vi "RSZVB Get Logical Port Common Ref Impedance.vi"(8 "error in (no error)":errorcluster {"code" format="%.0x"}, 9 "Port (1)":i32=1, 10 "Channel (1)":i32=1, 11 "VISA session":refnum<visa-resource-name>) -> (0 "error out":errorcluster {"code" format="%.0x"}, 1 "Imaginary":dbl format="%^.3e", 2 "Real":dbl format="%^.3e", 3 "dup VISA session":refnum<visa-resource-name>)   [LabVIEW 2011]
doc: "This VI returns the complex common mode reference impedance for the balanced (logical) port numbered <log_port>. \n\nRemote-control command(s):\n[SENSe<Ch>:]LPORt<log_port>:ZCOMmon?"
uses:
  _utility/RSZVB Global Data.vi
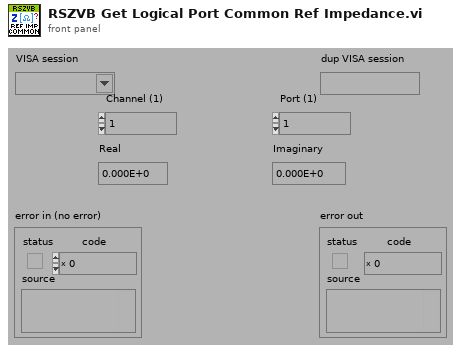
[diagram p1: front panel]
types:
  T1 = cluster{"Error Checking (T: On)":bool, "Installed Options":string[], "Data Valid?":bool, "Ports":i32, "Model":string[], "Option Checking (T: On)":bool}[]
  T2 = cluster{"Error Checking (T: On)":bool, "Installed Options":string[], "Data Valid?":bool, "Ports":i32, "Model":string[], "Option Checking (T: On)":bool}
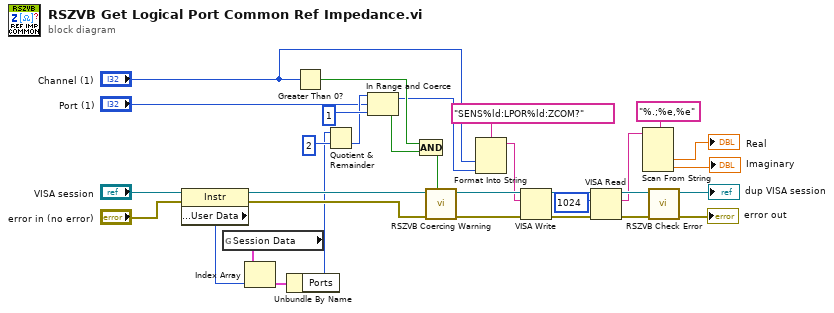
[diagram p0: block diagram]
diagram:
  n1 = property class="Instr"(reference="VISA session", error in="error in (no error)") -> (reference out=w31:refnum<visa-resource-name>, error out=w30:errorcluster, "General Settings:User Data"=w29:u32)
  n2 = global read "RSZVB Global Data.vi" "Session Data"() -> (w28:T1)
  n3 = Index Array(array=w28, index=w29) -> (element=w27:T2)
  n4 = Unbundle By Name(w27) -> ("Ports"=w23:i32)
  n5 = Greater Than 0?(x="Channel (1)") -> (x > 0?=w26:bool)
  n6 = Quotient & Remainder(x=w23, y=2) -> (floor(x/y)=w22:i32)  [unwired: 1 out]
  n7 = In Range and Coerce(upper limit=w22, x="Port (1)", lower limit=1) -> (coerced(x)=w16:i32, In Range?=w21:bool)
  n8 = Compound Arithmetic op=AND(w26, w21) -> (w25:bool)
  n9 = call "RSZVB Coercing Warning.vi"("In Range?"=w25, "error in (no error)"=w30, "VISA session"=w31) -> ("error out"=w20:errorcluster, "dup VISA session"=w19:refnum<visa-resource-name>)  [unwired: 7 in]
  n10 = Format Into String(format string="SENS%ld:LPOR%ld:ZCOM?", "Channel (1)", w16) -> (resulting string=w18:string)  [unwired: 2 in, 1 out]
  n11 = VISA Write(VISA resource name=w19, write buffer=w18, error in (no error)=w20) -> (VISA resource name out=w5:refnum<visa-resource-name>, error out=w6:errorcluster)  [unwired: 1 out]
  n12 = VISA Read(VISA resource name=w5, byte count=u32 1024 ("byte count (0)"), error in (no error)=w6) -> (VISA resource name out=w10:refnum<visa-resource-name>, read buffer=w7:string, error out=w9:errorcluster)  [unwired: 1 out]
  n13 = Scan From String(format string="%.;%e,%e", input string=w7) -> (output 1=→"Real":dbl, output 2=→"Imaginary":dbl)  [unwired: 4 in, 3 out]
  n14 = call "RSZVB Check Error.vi"("error in (no error)"=w9, "VISA session"=w10) -> ("error out"=→"error out":errorcluster, "dup VISA session"=→"dup VISA session":refnum<visa-resource-name>)  [unwired: 8 in]
